vi "gfitsio-write-comment.vi"(8 "error in (no error)":errorcluster, 9 "comment":string, 11 "gfits refnum":T1) -> (0 "error out":errorcluster, 3 "dup gfits refnum":T1)   [LabVIEW 2014, in "gfitsio.lvlib"]
doc: "Append a COMMENT keyword to the current HDU. The comment string will be continued over multiple keywords if it is longer than 70 characters."
uses:
  gfitsio.lvlib
  gfitsio-refnum.ctl
  gfitsio.dll
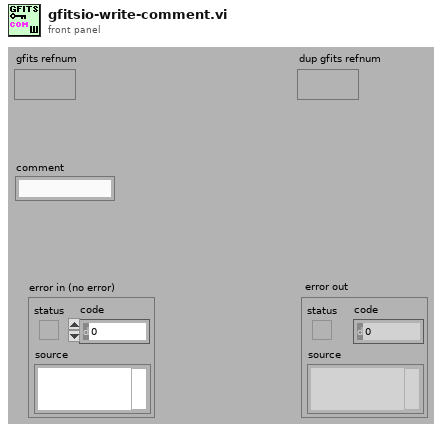
[diagram p1: front panel]
types:
  T1 = typedef "gfitsio.lvlib/gfitsio-refnum.ctl" = refnum<k1>
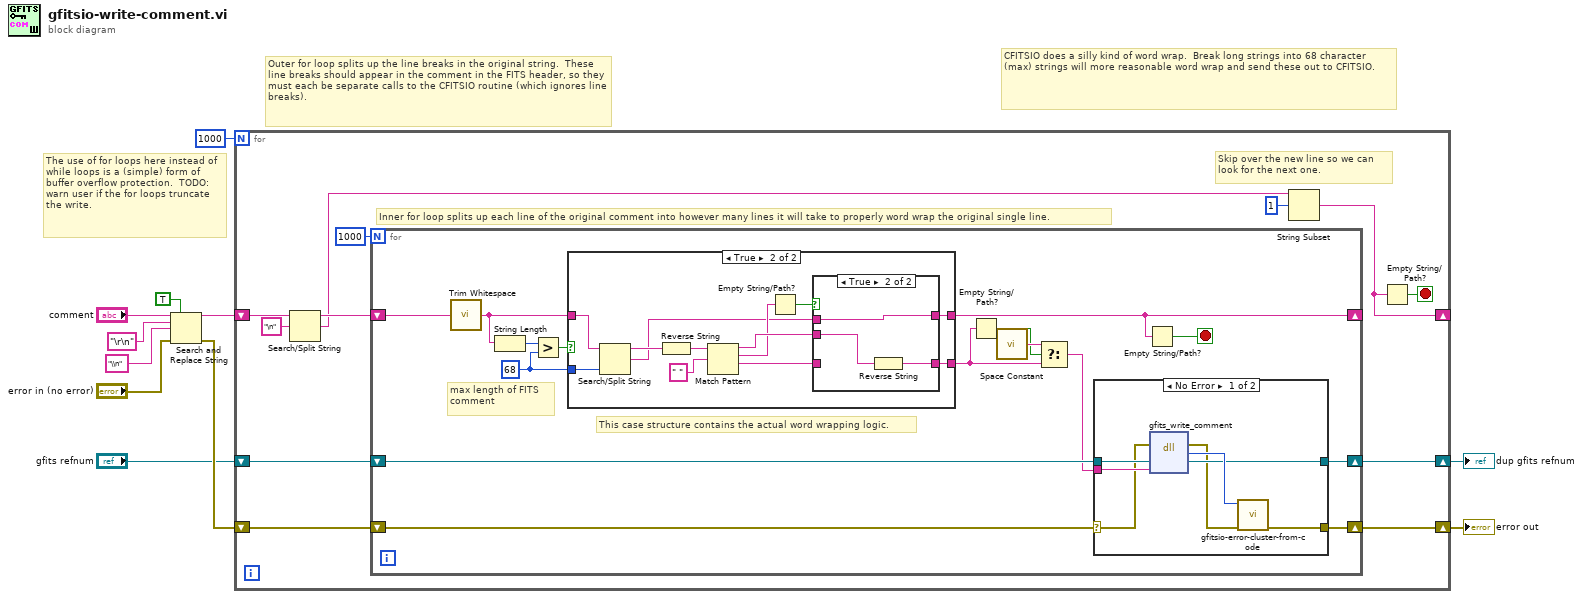
[diagram p0: block diagram]
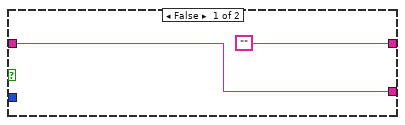
[diagram p3: hidden frame]
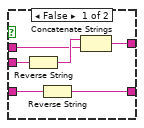
[diagram p4: hidden frame]
diagram:
  # "The use of for loops here instead of while loops is a (simple) form of buffer overflow protection.  TODO:  warn user if the for loops truncate the write."
  # "Outer for loop splits up the line breaks in the original string.  These line breaks should appear in the comment in the FITS header, so they must each be separate calls to the CFITSIO routine (which ignores line breaks)."
  # "CFITSIO does a silly kind of word wrap.  Break long strings into 68 character (max) strings will more reasonable word wrap and send these out to CFITSIO."
  n1 = Search and Replace String(replace all?=TRUE ("replace all? (F)"), input string="comment", search string="\r\n", replace string="\\n" ("replace string (\"\")"), error in="error in (no error)") -> (result string=w8:string, error out=w7:errorcluster)  [unwired: 3 in, 2 out]
  n2 = for {
    N: 1000 -> [_]
    shift-right: [w18] -> _
    shift-left: w8 -> [w23]
    shift-right: [w17] -> w3
    shift-left: "gfits refnum" -> [w16]
    shift-right: [w15] -> w4
    shift-left: w7 -> [w14]
    stop <- w13 stop-if-true
    # "Inner for loop splits up each line of the original comment into however many lines it will take to properly word wrap the original single line."
    # "Skip over the new line so we can look for the next one."
    n3 = Search/Split String(string=w23, search string/char (-)="\n" ("regular expression")) -> (substring before match=w21:string, match + rest of string=w19:string)  [unwired: 1 in, 1 out]
    n4 = for {
      N: 1000 -> [_]
      shift-right: [w38] -> _
      shift-left: w21 -> [w31]
      shift-right: [w27] -> w17
      shift-left: w16 -> [w26]
      shift-right: [w28] -> w15
      shift-left: w14 -> [w29]
      stop <- w24 stop-if-true
      w36 = 68 ("length (rest)")
      # "This case structure contains the actual word wrapping logic."
      # "max length of FITS comment"
      n5 = call <vilib>:"Trim Whitespace.vi"("string"=w31) -> ("trimmed string"=w30:string)  [unwired: 1 in]
      n6 = String Length(string=w30) -> (length=w37:i32)
      n7 = Greater?(x=w37, y=w36) -> (0:w35:bool)
      n8 = case shown="True" w35 {
        tunnel: ["" w56] -> w38
        tunnel: [w49 w52] -> w32
        tunnel: w30 -> [w49 w51]
        tunnel: w36 -> [_ w50]
        frame False {
        }
        frame True {
          n9 = Search/Split String(string=w51, offset (0)=w50) -> (substring before match=w58:string, match + rest of string=w55:string)  [unwired: 1 in, 1 out]
          n10 = Reverse String(1:w58) -> (0:w61:string)
          n11 = Match Pattern(string=w61, regular expression=" ") -> (before substring=w59:string, match substring=w57:string, after substring=w53:string)  [unwired: 1 in, 1 out]
          n12 = Empty String/Path?(string/path=w57) -> (empty?=w54:bool)
          n13 = case shown="True" w54 {
            tunnel: w59 -> [w67 w68]
            tunnel: [w65 w70] -> w56
            tunnel: w55 -> [w64 w70]
            tunnel: w53 -> [w63 _]
            tunnel: [w62 w69] -> w52
            frame False {
              n14 = Reverse String(1:w67) -> (0:w66:string)
              n15 = Reverse String(1:w63) -> (0:w62:string)
              n16 = Concatenate Strings(w66, w64) -> (w65:string)
            }
            frame True {
              n17 = Reverse String(1:w68) -> (0:w69:string)
            }
          }
        }
      }
      n18 = Empty String/Path?(string/path=w32) -> (empty?=w33:bool)
      n19 = call <vilib>:"Space Constant.vi"() -> ("String"=w34:string)
      n20 = Select(t=w34, s=w33, f=w32) -> (s? t:f=w25:string)
      n21 = case shown="No Error" w29 {
        selector: w29 -> [w40 w47]
        tunnel: [w44 w47] -> w28
        tunnel: w26 -> [w41 w46]
        tunnel: [w42 w46] -> w27
        tunnel: w25 -> [w43 _]
        frame No Error {
          n22 = dll-call lib="D:/optics_and_proj_related_stuff/labview_codes/gfitsio/gfitsio.dll" fn="gfits_write_comment"(error in=w40, "refnum"=w41, "comment"=w43) -> (error out=w39:errorcluster, "return type"=w45:i32, "refnum"=w42:T1)  [unwired: 3 in, 1 out]
          n23 = call "gfitsio-error-cluster-from-code.vi"("error in (no error)"=w39, "error code"=w45) -> ("error out"=w44:errorcluster)  [unwired: 9 out]
        }
        frame Error {
        }
      }
      n24 = Empty String/Path?(string/path=w38) -> (empty?=w24:bool)
    }
    n25 = String Subset(string=w19, offset (0)=1) -> (substring=w18:string)  [unwired: 1 in]
    n26 = Empty String/Path?(string/path=w18) -> (empty?=w13:bool)
  }
  "error out" <- w4
  "dup gfits refnum" <- w3
